vi "Write_sensor_power.vi"(7 "send to port (65500)":u16=65500, 8 "error in (no error)":errorcluster, 9 "ACK'd_clients addr":u32[](array[numeric]), 10 "IO expander data to write":u16, 11 "UDP Send Queue in":refnum<queue>) -> (0 "error out":errorcluster)   [LabVIEW 2013]
uses:
  UDP_read_datagram.ctl
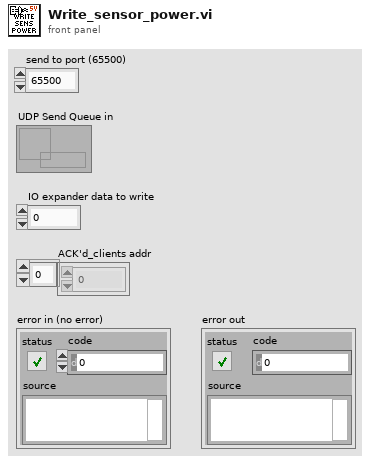
[diagram p1: front panel]
types:
  T1 = typedef "UDP_read_datagram.ctl" = cluster{"msg":string, "address":u32, "port":u16}
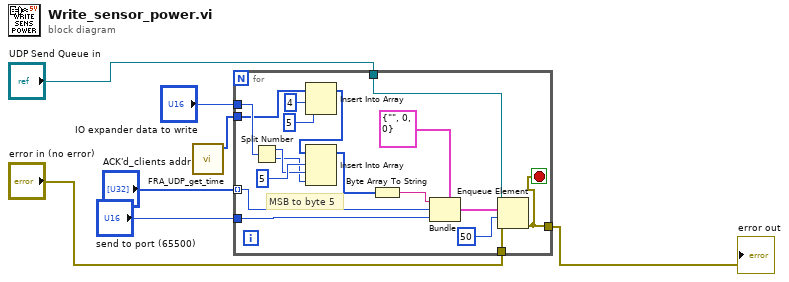
[diagram p0: block diagram]
diagram:
  n1 = call "FRA_UDP_get_time.vi"() -> ("array"=w5:u8[])  [unwired: 10 in, 1 out]
  n2 = for {
    tunnel: "ACK'd_clients addr" -> [w21] mode=indexing
    tunnel: "IO expander data to write" -> [w18]
    tunnel: "UDP Send Queue in" -> [w22]
    tunnel: "send to port (65500)" -> [w20]
    tunnel: w5 -> [w17]
    tunnel: "error in (no error)" -> [w11]
    tunnel: [w10] -> w7
    stop <- w10 stop-if-true
    # "MSB to byte 5"
    n3 = Split Number(x=w18) -> (hi(x)=w9:u8, lo(x)=w8:u8)
    n4 = Insert Into Array(array=w17, index=4, new element=u8 5 ("new element/subarray")) -> (w14:u8[])
    n5 = Insert Into Array(array=w14, index=5, new element #1=w9, new element #2=w8) -> (w12:u8[])
    n6 = Byte Array To String(unsigned byte array=w12) -> (string=w19:string)
    n7 = Bundle(cluster=T1 {"msg"="", "address"=0, "port"=0}, "msg"=w19, "address"=w21, "port"=w20) -> (w25:T1)
    n8 = Enqueue Element(queue=w22, element=w25, timeout in ms (-1)=50, error in (no error)=w11) -> (error out=w10:errorcluster)  [unwired: 2 out]
  }
  "error out" <- w7
